vi "Coincidence vs trigger level.vi"(7 "Reset latch":refnum<vi>, 8 "error in (no error)":errorcluster, 10 "Set VTrig":refnum<vi>, 11 "VTrig mV":refnum<vi>) -> (0 "Error out":errorcluster)   [LabVIEW 2016]
uses:
  <vilib>/Platform/TimedLoop/XDataNode/timing_clust.ctl
  <vilib>/Platform/TimedLoop/XDataNode/nitl_modes.ctl
  <vilib>/Platform/TimedLoop/XDataNode/wakeup.ctl
  <vilib>/platform/TimedLoop/XDataNode/XDataNode.xnode
  <vilib>/Platform/TimedLoop/XDataNode/XDNodeRunTimeDep.lvlib
  <vilib>/Analysis/NI_AALBase.lvlib
panel:
  out "Previous trigger level":dbl
  out "Trigger level increment":dbl
  out "Datapoints":i32
  out "Level number":i32
  out "Current\n trigger level":dbl
  in  "Datapoints per level":i32
  in  "finish level":bool
  in  "Recommended at 25C":bool
  in  "MPPC Bias":dbl
  in  "ROB ID":i32
  in  "MPPC Serial number":i32
  in  "Scintillator ID":i32
  in  "Data":i32[](array[numeric])
  out "Command Queue":string[](array[string])
  in  "stop":bool
  out "Histogram Graph":T1(graph)
  out "Waveform Chart":dbl(graph)
  in  "base path":path=path "C:/Users/install/Google Drive/CRT/Labview/CRT Controller Folder/VIs/Data taking/test2"
  in  "Levels":i32
  in  "Range min":i32 format="%.0f  mV"
  in  "Range max":i32 format="%.0f mV"
  in  "Begin characterization":bool
  in  "Period":i32=1000 format="%.0f ms"
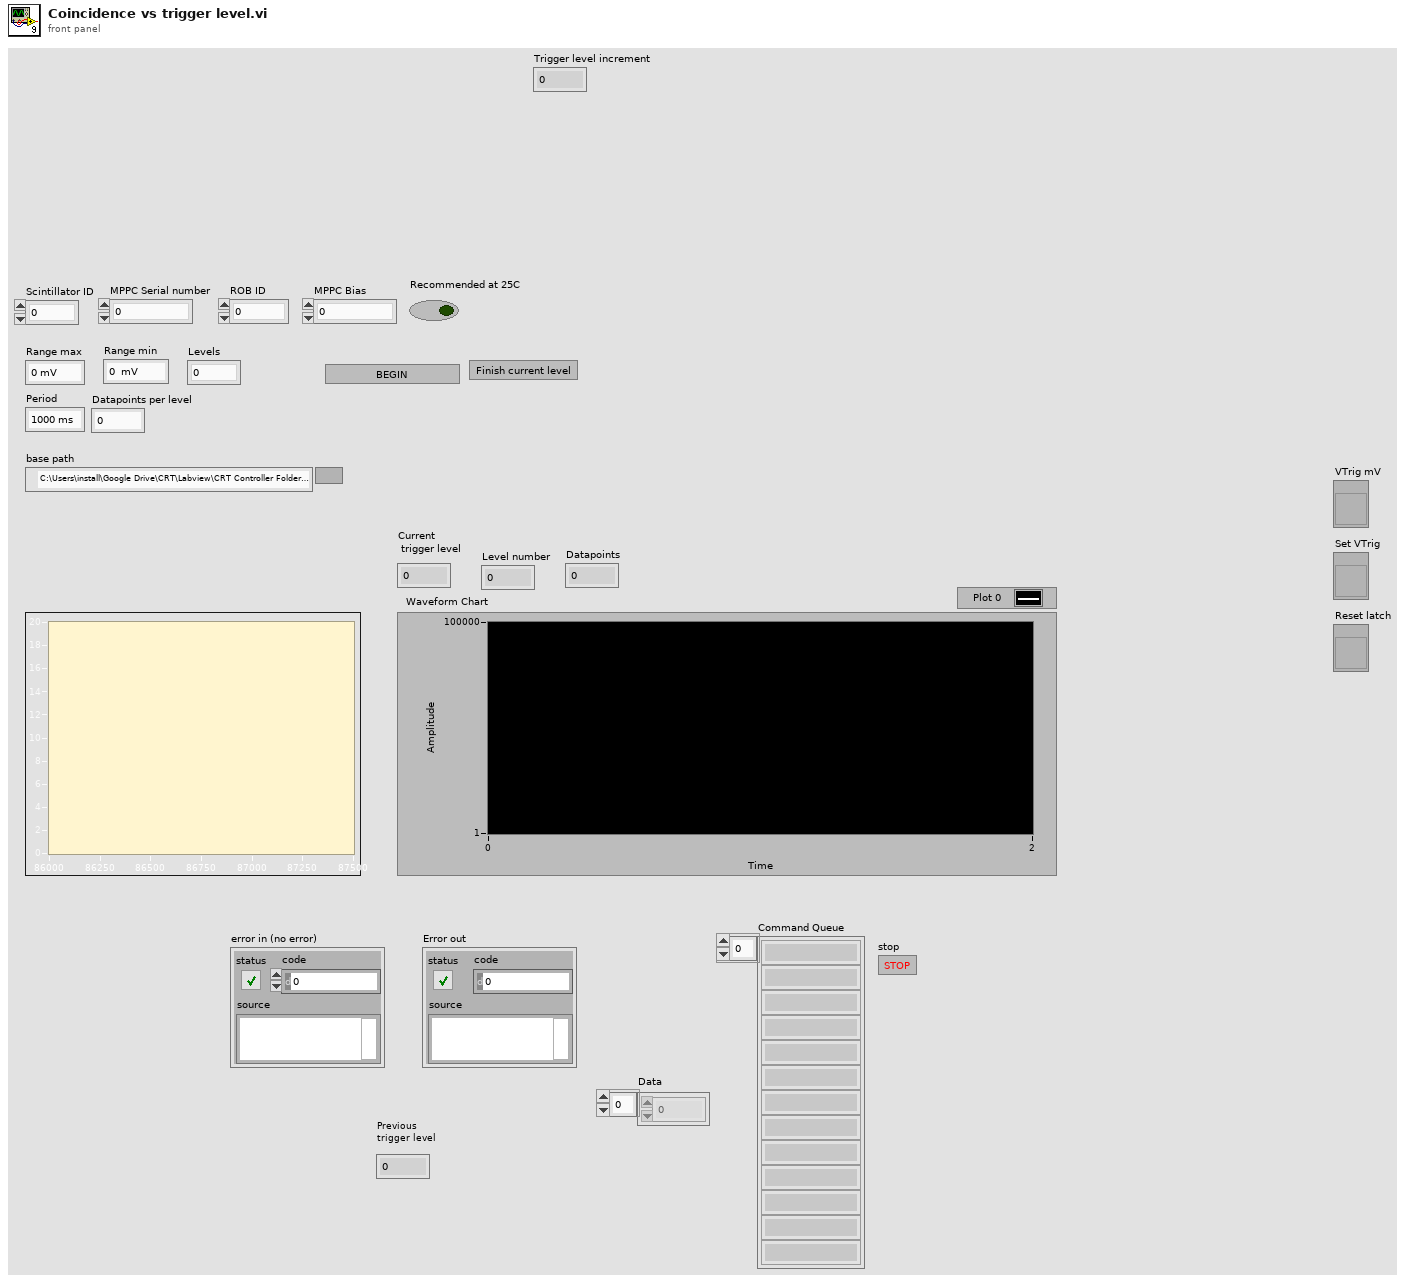
[diagram p1: front panel]
types:
  T1 = cluster{"X Values":dbl[], "Histogram: h(x)":i32[]}
  T2 = enum16{"open", "replace", "create", "open or create", "replace or create", "replace or create with confirmation"}
  T3 = enum16{"Reset", "ReadAndReset", "Read", "Add", "Init"}
  T4 = typedef "XDNodeRunTimeDep.lvlib/timing_clust.ctl" = cluster{"Expected End [f-1]":u64, "Actual End [f-1]":u64, "Finished Late? [f-1]":bool, "Expected End [i-1]":u64, "Actual End [i-1]":u64, "Finished Late? [i-1]":bool, "Expected Start [i]":u64, "Actual Start [i]":u64, "Expected Start [f]":u64, "Actual Start [f]":u64, "Source Name":string, "Structure Name":string, "Period":i64, "Deadline":i64, "Offset":i64, "Start":i64, "Priority":i32, "Timeout":i32, "Mode":T5, "Wakeup Reason":T6, "Error":errorcluster, "Source Type":string, "Secondary Source Type":string, "Global End Time":u64, "Global Start Time":u64, "Frame Duration":u64, "Iteration Duration":u64, "Assigned CPU":i32, "I/O Scan Engine Mode":u32}
  T5 = typedef "XDNodeRunTimeDep.lvlib/nitl_modes.ctl" = enum32{"No Change", "Process missed periods, maintain original phase", "Discard missed periods, maintain original phase", "Process missed periods, ignore original phase", "Discard missed periods, ignore original phase"}
  T6 = typedef "XDNodeRunTimeDep.lvlib/wakeup.ctl" = enum32{"Normal", "Aborted", "Asynchronous wakeup", "Timing source error", "Timed loop error", "Timeout"}
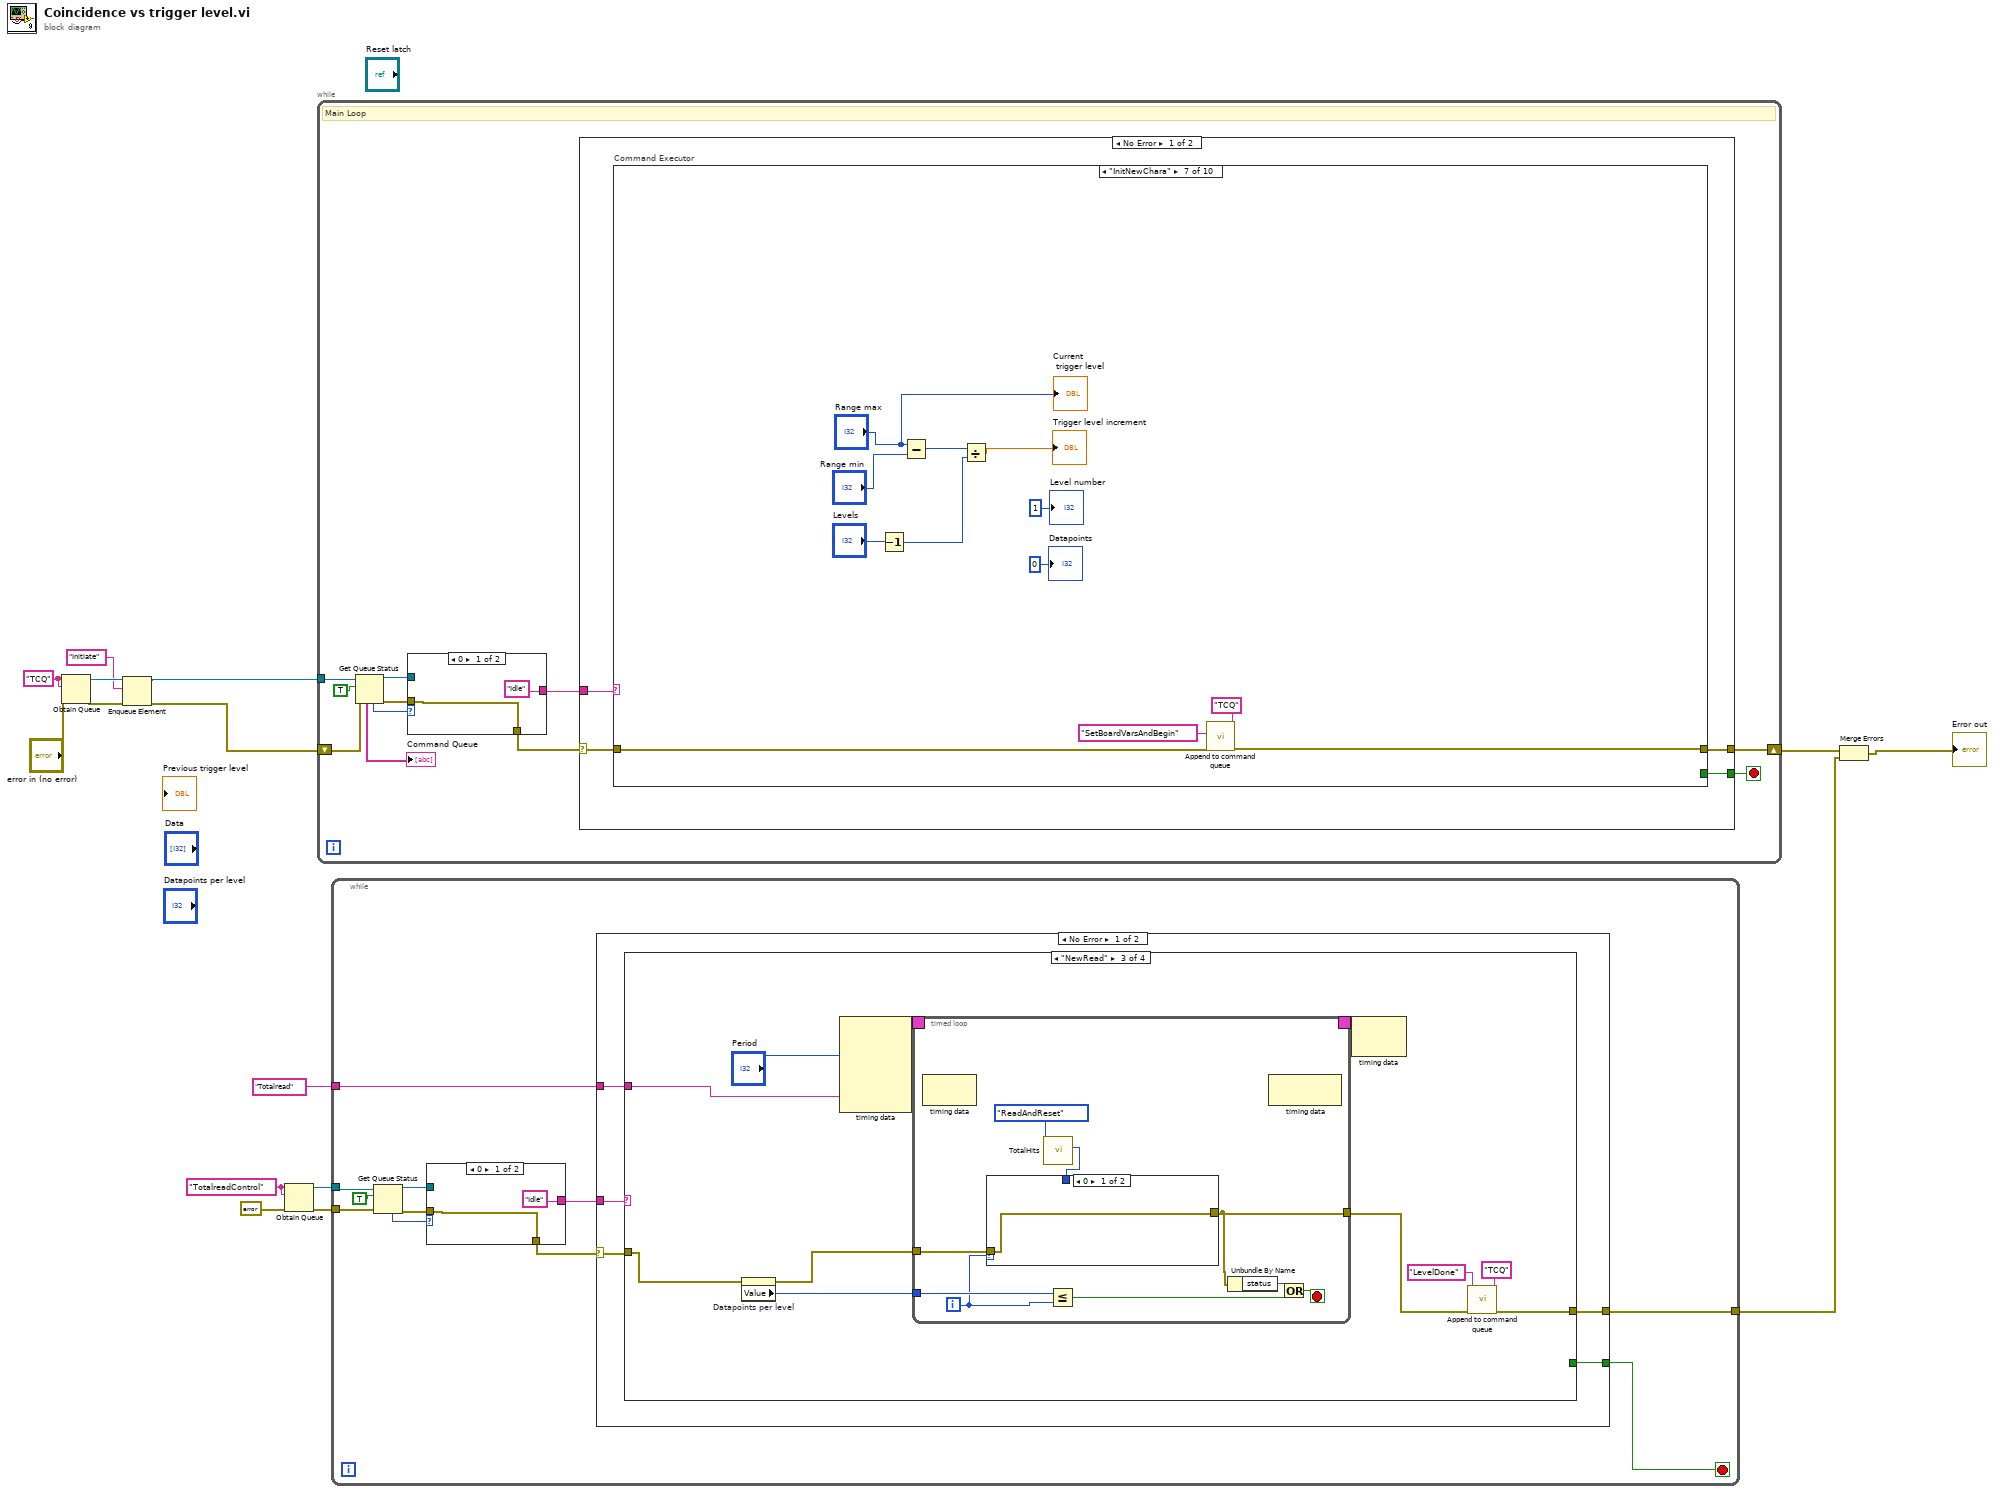
[diagram p0: block diagram]
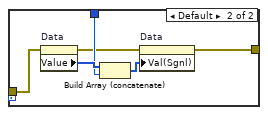
[diagram p4: hidden frame]
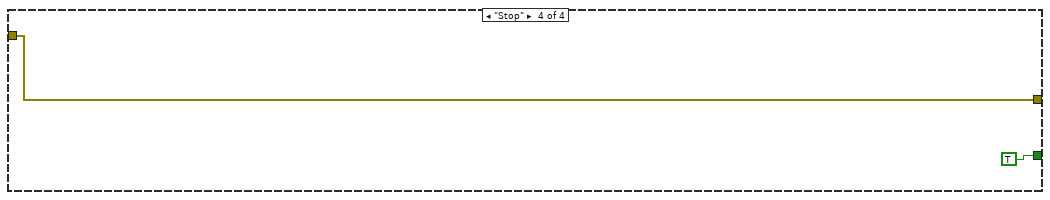
[diagram p5: hidden frame]
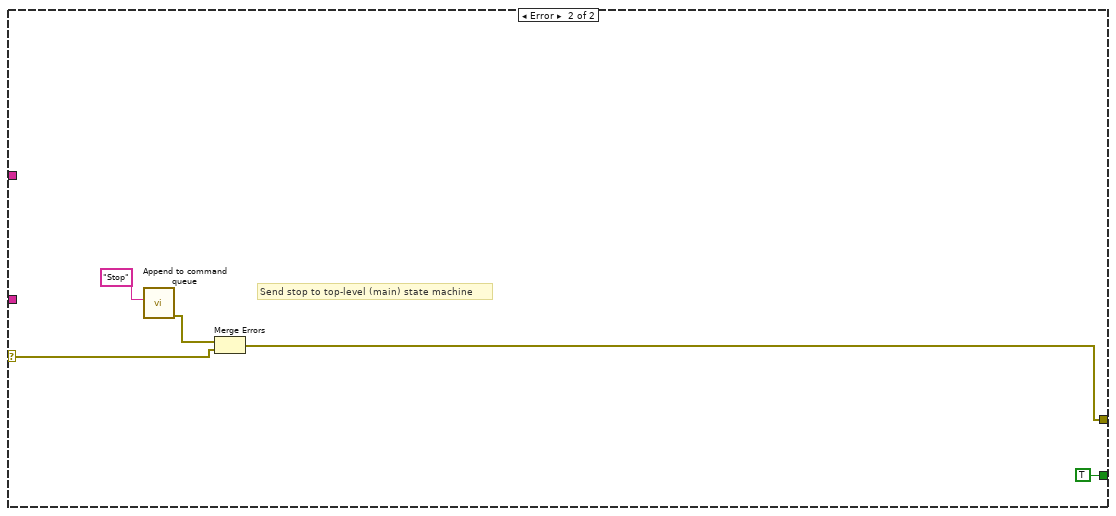
[diagram p6: hidden frame]
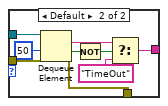
[diagram p7: hidden frame]
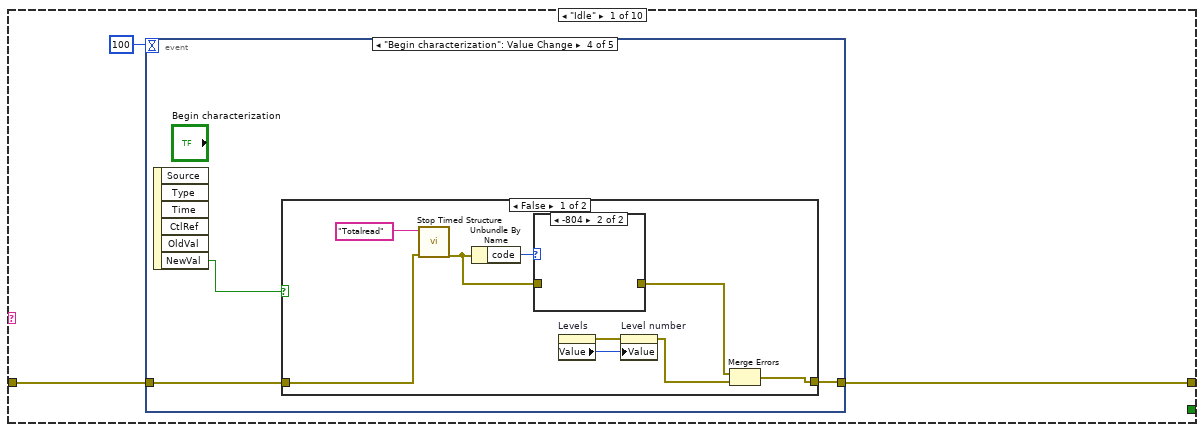
[diagram p8: hidden frame]
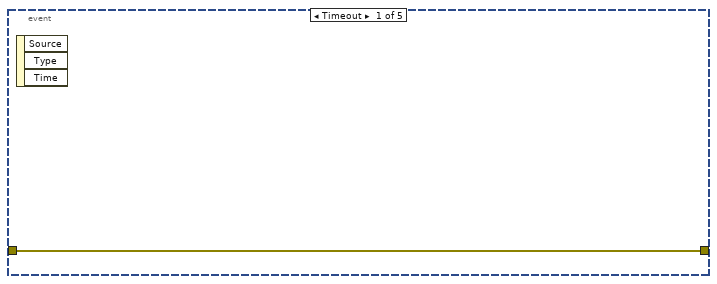
[diagram p9: hidden frame]
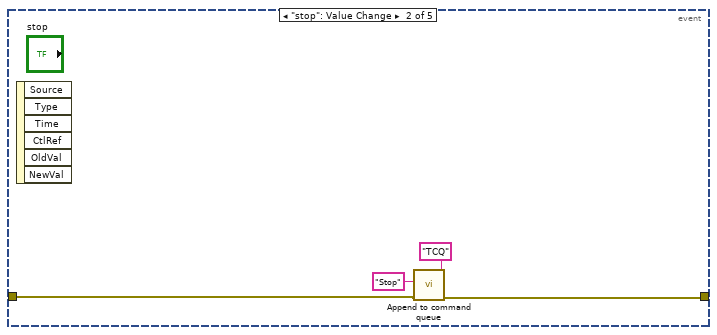
[diagram p10: hidden frame]
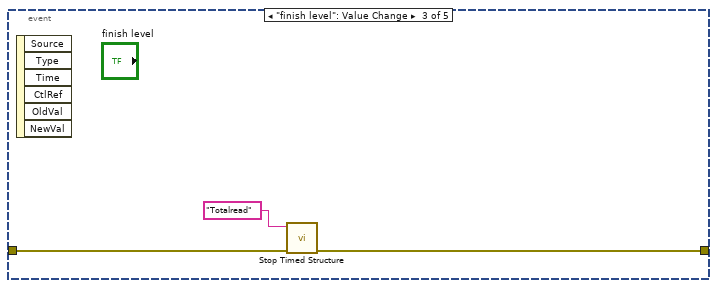
[diagram p11: hidden frame]
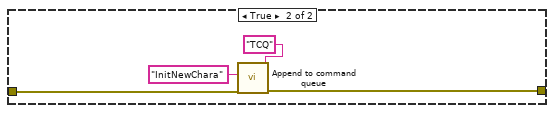
[diagram p13: hidden frame]
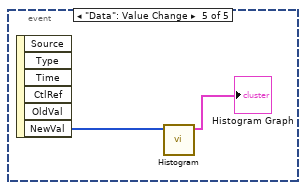
[diagram p14: hidden frame]
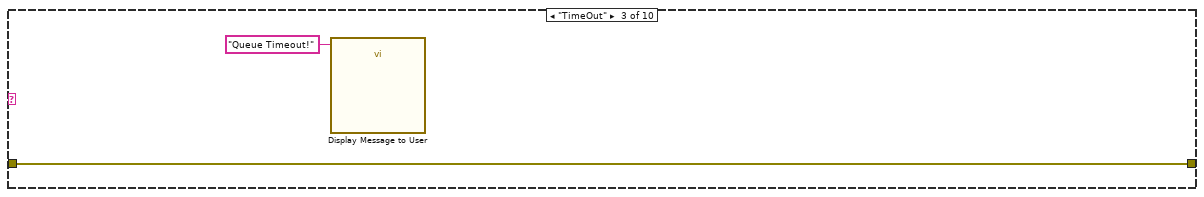
[diagram p16: hidden frame]
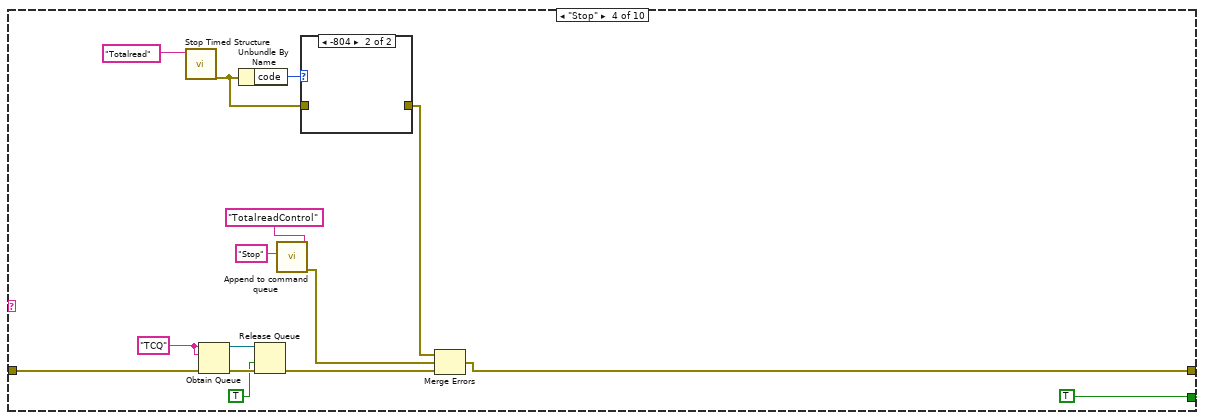
[diagram p17: hidden frame]
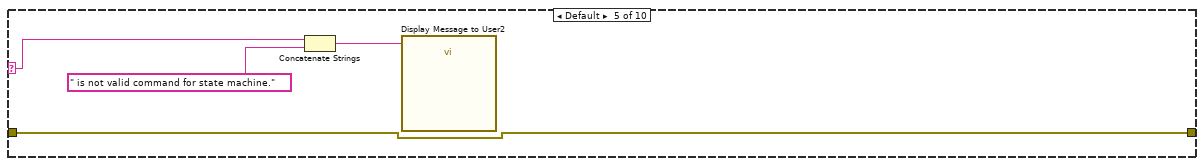
[diagram p19: hidden frame]
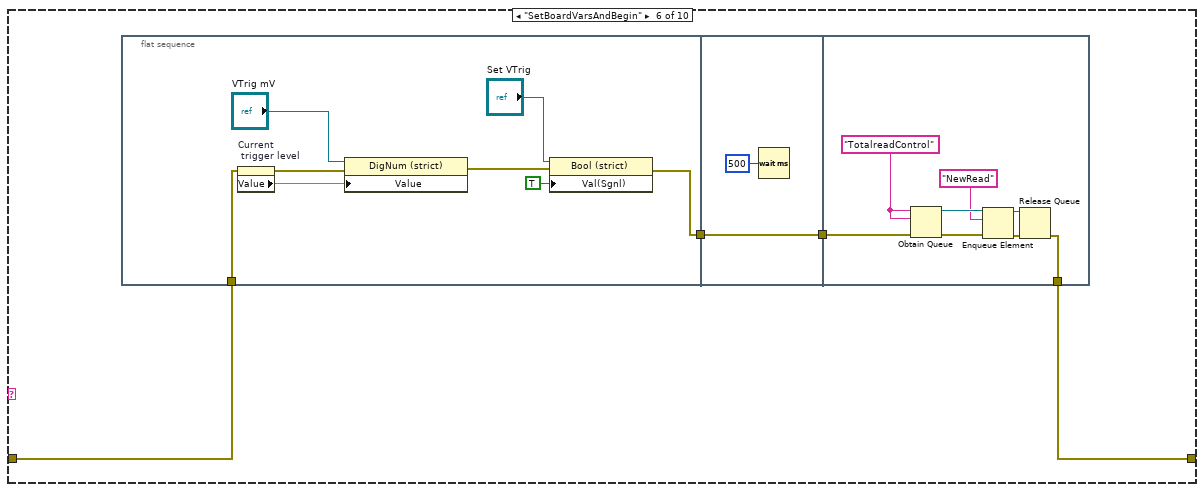
[diagram p20: hidden frame]
diagram:
  w7 = "TotalreadControl" ("name (unnamed)")
  w15 = "TCQ" ("name (unnamed)")
  n1 = Obtain Queue(name (unnamed)=w15, element data type=w15, error in (no error)="error in (no error)") -> (queue out=w13:refnum<queue>, error out=w11:errorcluster)  [unwired: 2 in, 1 out]
  n2 = Enqueue Element(queue=w13, element="Initiate", error in (no error)=w11) -> (queue out=w4:refnum<queue>, error out=w10:errorcluster)  [unwired: 1 in, 1 out]
  n3 = Obtain Queue(name (unnamed)=w7, element data type=w7, error in (no error)=errorcluster {"status"=FALSE, "code"=0, "source"=""}) -> (queue out=w6:refnum<queue>, error out=w5:errorcluster)  [unwired: 2 in, 1 out]
  n4 = while {
    tunnel: w4 -> [w22]
    shift-right: [w18] -> w3
    shift-left: w10 -> [w19]
    stop <- w17 stop-if-true
    # "Main Loop"
    n5 = Get Queue Status(queue=w22, return elements? (F)=TRUE, error in (no error)=w19) -> (queue out=w25:refnum<queue>, error out=w24:errorcluster, # elements in queue=w26:i32, elements=→"Command Queue":string[])  [unwired: 4 out]
    n6 = case shown="0" w26 {
      tunnel: ["Idle" ("element") w254] -> w20
      tunnel: w25 -> [_ w260]
      tunnel: w24 -> [w250 w259]
      tunnel: [w250 w253] -> w16
      frame 0 {
      }
      frame Default {
        n7 = Dequeue Element(queue=w260, timeout in ms (-1)=50, error in (no error)=w259) -> (element=w258:string, timed out?=w257:bool, error out=w253:errorcluster)  [unwired: 1 out]
        n8 = Not(x=w257) -> (.not. x?=w256:bool)
        n9 = Select(t=w258, s=w256, f="TimeOut") -> (s? t:f=w254:string)
      }
    }
    n10 = case shown="No Error" w16 {
      selector: w16 -> [w27 w242]
      tunnel: w20 -> [w30 _]
      tunnel: [w29 w241] -> w18
      tunnel: [w28 TRUE] -> w17
      frame No Error {
        n11 = case "Command Executor" shown="\"InitNewChara\"" w30 {
          selector: w30 -> [_ _ _ _ w81 _ _ _ _ _]
          tunnel: [w31 w61 w62 w64 w80 w84 w109 w125 w162 w227] -> w29
          tunnel: w27 -> [w32 w61 w62 w73 w80 w87 w110 w127 w164 w229]
          tunnel: [_ _ _ TRUE _ _ _ _ _ _] -> w28
          frame "Idle" {
            n12 = event shown="[3] \"Begin characterization\": Value Change" {
              selector: _ -> [_ _ _ _ _]
              dyn-events: _ -> [_ _ _ _ _]
              timeout: 100 -> [_ _ _ _ _]
              tunnel: w32 -> [w34 w38 w41 w44 _]
              tunnel: [w34 w37 w40 w43 _] -> w31
              event Timeout {
                n13 = event-data() -> ()  [unwired: 1 in, 3 out]
              }
              event "stop": Value Change {
                n14 = event-data() -> ()  [unwired: 1 in, 6 out]
                n15 = call "Append to command queue.vi"("Name (CommandQueue)"="TCQ", "error in (no error)"=w38, "Single command"="Stop") -> ("error out"=w37:errorcluster)  [unwired: 8 in]
              }
              event "finish level": Value Change {
                n16 = event-data() -> ()  [unwired: 1 in, 6 out]
                n17 = call <vilib>:"Stop Timed Structure.vi"("error in (no error)"=w41, "name"="Totalread" ("Structure Name")) -> ("error out"=w40:errorcluster)  [unwired: 9 in]
              }
              event "Begin characterization": Value Change {
                n18 = event-data() -> ("NewVal"=w42:bool)  [unwired: 1 in, 5 out]
                n19 = case shown="False" w42 {
                  tunnel: w44 -> [w48 w57]
                  tunnel: [w46 w56] -> w43
                  frame False {
                    n20 = call <vilib>:"Stop Timed Structure.vi"("error in (no error)"=w48, "name"="Totalread" ("Structure Name")) -> ("error out"=w49:errorcluster)  [unwired: 9 in]
                    n21 = Unbundle By Name(w49) -> ("code"=w50:i32)
                    n22 = case shown="-804" w50 {
                      tunnel: w49 -> [w54 _]
                      tunnel: [w54 _] -> w45
                      frame Default {
                      }
                      frame -804 {
                      }
                    }
                    n23 = property on="Levels" class="DigNum (strict)"() -> (error out=w52:errorcluster, "Value"=w53:i32)  [unwired: 2 in, 1 out]
                    n24 = property on="Level number" class="DigNum (strict)"(error in=w52, "Value"=w53) -> (error out=w47:errorcluster)  [unwired: 1 in, 1 out]
                    n25 = Merge Errors(w45, w47) -> (w46:errorcluster)
                  }
                  frame True {
                    n26 = call "Append to command queue.vi"("Name (CommandQueue)"="TCQ", "error in (no error)"=w57, "Single command"="InitNewChara") -> ("error out"=w56:errorcluster)  [unwired: 8 in]
                  }
                }
              }
              event "Data": Value Change {
                n27 = event-data() -> ("NewVal"=w59:i32[])  [unwired: 1 in, 5 out]
                n28 = call <vilib>:"Histogram.vi"("X"=w59) -> ("Histogram Graph"=→"Histogram Graph":T1)  [unwired: 7 in, 3 out]
              }
            }
          }
          frame "Initiate" {
          }
          frame "TimeOut" {
            n29 = call "Display Message to User"("Message"="Queue Timeout!" ("string")) -> ()  [unwired: 9 in, 2 out]
          }
          frame "Stop" {
            w74 = "TCQ" ("name (unnamed)")
            n30 = call <vilib>:"Stop Timed Structure.vi"("name"="Totalread" ("Structure Name")) -> ("error out"=w66:errorcluster)  [unwired: 10 in]
            n31 = Obtain Queue(name (unnamed)=w74, element data type=w74, error in (no error)=w73) -> (queue out=w77:refnum<queue>, error out=w76:errorcluster)  [unwired: 2 in, 1 out]
            n32 = Unbundle By Name(w66) -> ("code"=w69:i32)
            n33 = Release Queue(queue=w77, force destroy? (F)=TRUE, error in (no error)=w76) -> (error out=w67:errorcluster)  [unwired: 2 out]
            n34 = call "Append to command queue.vi"("Name (CommandQueue)"="TotalreadControl", "Single command"="Stop") -> ("error out"=w68:errorcluster)  [unwired: 9 in]
            n35 = case shown="-804" w69 {
              tunnel: w66 -> [w79 _]
              tunnel: [w79 _] -> w65
              frame Default {
              }
              frame -804 {
              }
            }
            n36 = Merge Errors(w65, w68, w67) -> (w64:errorcluster)
          }
          frame Default {
            n37 = Concatenate Strings(w81, " is not valid command for state machine." ("string")) -> (w82:string)
            n38 = call "Display Message to User2"("Message"=w82) -> ()  [unwired: 9 in, 2 out]
          }
          frame "SetBoardVarsAndBegin" {
            n39 = flat-sequence {
              tunnel: w87 -> [w89]
              tunnel: [w88] -> w86
              tunnel: w86 -> [w96]
              tunnel: [w96] -> w85
              tunnel: w85 -> [w100]
              tunnel: [w99] -> w84
              frame #0 {
                n40 = property on="Current\n trigger level" class="DigNum (strict)"(error in=w89) -> (error out=w91:errorcluster, "Value"=w92:dbl)  [unwired: 1 in, 1 out]
                n41 = property class="DigNum (strict)"(reference="VTrig mV", error in=w91, "Value"=w92) -> (error out=w90:errorcluster)  [unwired: 1 out]
                n42 = property class="Bool (strict)"(reference="Set VTrig", error in=w90, "Val(Sgnl)"=TRUE ("Value (Signaling)")) -> (error out=w88:errorcluster)  [unwired: 1 out]
              }
              frame #1 {
                n43 = Wait (ms)(milliseconds to wait=u32 500) -> ()  [unwired: 1 out]
              }
              frame #2 {
                w101 = "TotalreadControl" ("name (unnamed)")
                n44 = Obtain Queue(name (unnamed)=w101, element data type=w101, error in (no error)=w100) -> (queue out=w105:refnum<queue>, error out=w104:errorcluster)  [unwired: 2 in, 1 out]
                n45 = Enqueue Element(queue=w105, element="NewRead", error in (no error)=w104) -> (queue out=w102:refnum<queue>, error out=w103:errorcluster)  [unwired: 1 in, 1 out]
                n46 = Release Queue(queue=w102, error in (no error)=w103) -> (error out=w99:errorcluster)  [unwired: 1 in, 2 out]
              }
            }
          }
          frame "InitNewChara" {
            n47 = Decrement(x="Levels") -> (x-1=w106:i32)
            n48 = Subtract(x="Range max", y="Range min") -> (x-y=w115:i32)
            n49 = Divide(x=w115, y=w106) -> (x/y=→"Trigger level increment":dbl)
            n50 = call "Append to command queue.vi"("Name (CommandQueue)"="TCQ", "error in (no error)"=w110, "Single command"="SetBoardVarsAndBegin") -> ("error out"=w109:errorcluster)  [unwired: 8 in]
            "Current\n trigger level" <- "Range max"
            "Level number" <- 1 ("Level number")
            "Datapoints" <- 0 ("Datapoints")
          }
          frame "LevelDone" {
            n51 = property on="Levels" class="DigNum (strict)"(error in=w127) -> (error out=w128:errorcluster, "Value"=w129:i32)  [unwired: 1 in, 1 out]
            n52 = property on="Level number" class="DigNum (strict)"(error in=w128) -> (error out=w122:errorcluster, "Value"=w130:i32)  [unwired: 1 in, 1 out]
            n53 = Equal?(x=w130, y=w129) -> (x = y?=w126:bool)
            n54 = call "Append to command queue.vi"("Name (CommandQueue)"="TCQ", "error in (no error)"=w122, "Single command"="SaveData") -> ("error out"=w119:errorcluster)  [unwired: 8 in]
            n55 = property on="Current\n trigger level" class="DigNum (strict)"(error in=w119) -> (error out=w120:errorcluster, "Value"=w121:dbl)  [unwired: 1 in, 1 out]
            n56 = property on="Previous trigger level" class="DigNum (strict)"(error in=w120, "Value"=w121) -> (error out=w118:errorcluster)  [unwired: 1 in, 1 out]
            n57 = case shown="False" w126 {
              tunnel: w118 -> [w136 w147]
              tunnel: [w133 w146] -> w125
              frame False {
                n58 = property on="Trigger level increment" class="DigNum (strict)"(error in=w136) -> (error out=w141:errorcluster, "Value"=w140:dbl)  [unwired: 1 in, 1 out]
                n59 = property on="Current\n trigger level" class="DigNum (strict)"(error in=w141) -> (error out=w138:errorcluster, "Value"=w131:dbl)  [unwired: 1 in, 1 out]
                n60 = Subtract(x=w131, y=w140) -> (x-y=w139:dbl)
                n61 = property on="Current\n trigger level" class="DigNum (strict)"(error in=w138, "Value"=w139) -> (error out=w137:errorcluster)  [unwired: 1 in, 1 out]
                n62 = property on="Level number" class="DigNum (strict)"(error in=w137) -> (error out=w142:errorcluster, "Value"=w144:i32)  [unwired: 1 in, 1 out]
                n63 = Increment(x=w144) -> (x+1=w143:i32)
                n64 = property on="Level number" class="DigNum (strict)"(error in=w142, "Value"=w143) -> (error out=w132:errorcluster)  [unwired: 1 in, 1 out]
                n65 = call "Append to command queue.vi"("Name (CommandQueue)"="TCQ", "error in (no error)"=w132, "Single command"="SetBoardVarsAndBegin") -> ("error out"=w133:errorcluster)  [unwired: 8 in]
              }
              frame True {
                n66 = call "Append to command queue.vi"("Name (CommandQueue)"="TCQ", "error in (no error)"=w147, "Single command"="Reset") -> ("error out"=w146:errorcluster)  [unwired: 8 in]
              }
            }
          }
          frame "SaveData" {
            w153 = "\t"
            n67 = control-ref of="Period"() -> (w203:refnum<vi>)
            n68 = control-ref of="Previous trigger level"() -> (w156:refnum<vi>)
            n69 = property class="DigNum (strict)"(reference=w203, error in=w164) -> (error out=w189:errorcluster, "Value"=w172:i32)  [unwired: 1 out]
            n70 = property class="DigNum (strict)"(reference=w156, error in=w189) -> (error out=w188:errorcluster, "Value"=w204:dbl)  [unwired: 1 out]
            n71 = property on="Data" class="Arr (strict)"(error in=w188) -> (error out=w187:errorcluster, "Value"=w171:i32[])  [unwired: 1 in, 1 out]
            n72 = property on="base path" class="Path"(error in=w164) -> (error out=w163:errorcluster, "Value"=w185:path)  [unwired: 1 in, 1 out]
            n73 = Build Path(base path=w185, name or relative path="Summary.csv") -> (appended path=w180:path)
            n74 = Number To Decimal String(number=w204) -> (decimal integer string=w168:string)  [unwired: 1 in]
            n75 = Number To Decimal String(number=w172) -> (decimal integer string=w155:string)  [unwired: 1 in]
            n76 = Open/Create/Replace File(file path (use dialog)=w180, error in=w163, operation (0:open)=T2."open") -> (refnum out=w183:refnum<file>, error out=w182:errorcluster)  [unwired: 3 in, 1 out]
            n77 = Unbundle By Name(w182) -> ("code"=w181:i32)
            n78 = Concatenate Strings(w168, "mV " ("string"), w155, "s.csv " ("string")) -> (w202:string)
            n79 = Array To Spreadsheet String(delimiter (Tab)="\r\n", array=w171, 3:"%d" ("format string")) -> (spreadsheet string=w195:string)
            n80 = Build Path(base path="base path", name or relative path=w202) -> (appended path=w207:path)
            n81 = call "Build header single level.vi"("Overvoltage"="MPPC Bias", "Recommended at 25C"="Recommended at 25C", "MPPC Serial number"="MPPC Serial number", "ROB ID"="ROB ID", "Scintillator ID"="Scintillator ID") -> ("Header"=w179:string)  [unwired: 6 in]
            n82 = case shown="7" w181 {
              tunnel: w183 -> [_ w226]
              tunnel: w182 -> [_ w225]
              tunnel: w180 -> [w218 _]
              tunnel: w179 -> [w213 _]
              tunnel: [w215 w221] -> w173
              tunnel: [w214 w220] -> w174
              frame 7 {
                n83 = Open/Create/Replace File(file path (use dialog)=w218, operation (0:open)=T2."create") -> (refnum out=w216:refnum<file>, error out=w217:errorcluster)  [unwired: 4 in, 1 out]
                n84 = Concatenate Strings(w213, "Trigger\tmean\tstandard deviation\tvariance\tpool size\tperiod" ("delimiter (Tab)"), "\r\n") -> (w211:string)
                n85 = Write to Text File(file (use dialog)=w216, text=w211, error in=w217) -> (refnum out=w215:refnum<file>, error out=w214:errorcluster)  [unwired: 1 in, 1 out]
              }
              frame Default {
                n86 = Get File Size(file=w226, error in=w225) -> (refnum out=w224:refnum<file>, size (in bytes)=w223:i64, 0:w222:errorcluster)
                n87 = Set File Position(offset (in bytes) (0)=w223, refnum=w224, error in=w222) -> (refnum out=w221:refnum<file>, error out=w220:errorcluster)  [unwired: 1 in]
              }
            }
            n88 = Concatenate Strings(w179, w195) -> (w192:string)
            n89 = Open/Create/Replace File(file path (use dialog)=w207, error in=w187, operation (0:open)=T2."open or create") -> (refnum out=w194:refnum<file>, error out=w193:errorcluster)  [unwired: 3 in, 1 out]
            n90 = call <vilib>:"Std Deviation and Variance.vi"("X"=w171) -> ("mean"=w157:dbl, "standard deviation"=w178:dbl, "variance"=w177:dbl)  [unwired: 1 in]
            "Waveform Chart" <- w157
            n91 = Array Size(array=w171) -> (size(s)=w170:i32)
            n92 = Build Array(w157, w178, w177) -> (w175:dbl[])
            n93 = Number To Decimal String(number=w170) -> (decimal integer string=w167:string)  [unwired: 1 in]
            n94 = Write to Text File(file (use dialog)=w194, text=w192, error in=w193) -> (refnum out=w191:refnum<file>, error out=w190:errorcluster)  [unwired: 1 in, 1 out]
            n95 = Array To Spreadsheet String(array=w175, 3:"%5.3f" ("format string")) -> (spreadsheet string=w152:string)  [unwired: 1 in]
            n96 = Close File(refnum=w191, error in=w190) -> (error out=w160:errorcluster)  [unwired: 1 out]
            n97 = Search/Split String(string=w152, search string/char (-)="\r\n") -> (substring before match=w150:string)  [unwired: 1 in, 2 out]
            n98 = Concatenate Strings(w168, w153, w150, w153, w167, w153, w155, "\r\n") -> (w169:string)
            n99 = Write to Text File(file (use dialog)=w173, text=w169, error in=w174) -> (refnum out=w165:refnum<file>, error out=w166:errorcluster)  [unwired: 1 in, 1 out]
            n100 = property on="Data" class="Arr (strict)"(error in=w160, "Value"=i32[] [] ("Data")) -> (error out=w159:errorcluster)  [unwired: 1 in, 1 out]
            n101 = Close File(refnum=w165, error in=w166) -> (error out=w161:errorcluster)  [unwired: 1 out]
            n102 = Merge Errors(w161, w159) -> (w162:errorcluster)
          }
          frame "Reset" {
            n103 = property on="Level number" class="DigNum (strict)"(error in=w229, "Value"=1 ("Level number")) -> (error out=w228:errorcluster)  [unwired: 1 in, 1 out]
            n104 = property on="Datapoints" class="DigNum (strict)"(error in=w228, "Value"=0 ("Datapoints")) -> (error out=w227:errorcluster)  [unwired: 1 in, 1 out]
          }
        }
      }
      frame Error {
        w244 = "TCQ" ("name (unnamed)")
        n105 = call <vilib>:"Stop Timed Structure.vi"("name"="Totalread" ("Structure Name")) -> ("error out"=w233:errorcluster)  [unwired: 10 in]
        n106 = Obtain Queue(name (unnamed)=w244, element data type=w244) -> (queue out=w247:refnum<queue>, error out=w246:errorcluster)  [unwired: 3 in, 1 out]
        n107 = Unbundle By Name(w233) -> ("code"=w234:i32)
        n108 = call "Append to command queue.vi"("Single command"="Stop") -> ("error out"=w239:errorcluster)  [unwired: 10 in]
        n109 = Release Queue(queue=w247, force destroy? (F)=TRUE, error in (no error)=w246) -> (error out=w243:errorcluster)  [unwired: 2 out]
        n110 = case shown="-804" w234 {
          tunnel: w233 -> [w249 _]
          tunnel: [w249 _] -> w232
          frame Default {
          }
          frame -804 {
          }
        }
        n111 = call "Append to command queue.vi"("Name (CommandQueue)"="TotalreadControl", "Single command"="Stop") -> ("error out"=w236:errorcluster)  [unwired: 9 in]
        n112 = Merge Errors(w232, w236, w239, w243, w242) -> (w241:errorcluster)
      }
    }
  }
  n113 = while {
    tunnel: "Totalread" ("Structure Name") -> [w271]
    tunnel: w6 -> [w266]
    tunnel: w5 -> [w265]
    tunnel: [w262] -> w2
    stop <- w261 stop-if-true
    n114 = Get Queue Status(queue=w266, return elements? (F)=TRUE, error in (no error)=w265) -> (queue out=w269:refnum<queue>, error out=w268:errorcluster, # elements in queue=w270:i32)  [unwired: 5 out]
    n115 = case shown="0" w270 {
      tunnel: ["Idle" ("element") w324] -> w264
      tunnel: w269 -> [_ w330]
      tunnel: w268 -> [w320 w329]
      tunnel: [w320 w323] -> w263
      frame 0 {
      }
      frame Default {
        n116 = Dequeue Element(queue=w330, timeout in ms (-1)=50, error in (no error)=w329) -> (element=w328:string, timed out?=w327:bool, error out=w323:errorcluster)  [unwired: 1 out]
        n117 = Not(x=w327) -> (.not. x?=w326:bool)
        n118 = Select(t=w328, s=w326, f="TimeOut") -> (s? t:f=w324:string)
      }
    }
    n119 = case shown="No Error" w263 {
      selector: w263 -> [w274 w317]
      tunnel: w271 -> [w276 _]
      tunnel: w264 -> [w275 _]
      tunnel: [w273 w316] -> w262
      tunnel: [w272 TRUE] -> w261
      frame No Error {
        n120 = case shown="\"NewRead\"" w275 {
          tunnel: w276 -> [_ _ w289 _]
          tunnel: [w277 w278 w288 w314] -> w273
          tunnel: w274 -> [w277 w278 w287 w314]
          tunnel: [_ _ _ TRUE] -> w272
          frame "TimeOut" {
          }
          frame Default {
          }
          frame "NewRead" {
            n121 = property on="Datapoints per level" class="DigNum (strict)"(error in=w287) -> (error out=w280:errorcluster, "Value"=w279:i32)  [unwired: 1 in, 1 out]
            n122 = node-c288("Period", w289) -> (w286:T4)  [unwired: 3 in]
            n123 = timed-loop {
              timing: w286 -> [_]
              timing-out: [_] -> w285
              tunnel: w280 -> [w296]
              tunnel: [w294] -> w281
              tunnel: w279 -> [w295]
              i -> [w290]
              stop <- w291 stop-if-true
              n124 = node-c288() -> ()  [unwired: 1 in, 1 out]
              n125 = call "TotalHits.vi"("Action"=T3."ReadAndReset") -> ("Result"=w297:u64)  [unwired: 10 in]
              n126 = case shown="0" w290 {
                tunnel: w297 -> [_ w304]
                tunnel: w296 -> [w299 w301]
                tunnel: [w299 w300] -> w294
                frame 0 {
                }
                frame Default {
                  n127 = property on="Data" class="Arr (strict)"(error in=w301) -> (error out=w302:errorcluster, "Value"=w305:i32[])  [unwired: 1 in, 1 out]
                  n128 = Build Array (concatenate)(w305, w304) -> (w303:u64[])
                  n129 = property on="Data" class="Arr (strict)"(error in=w302, "Val(Sgnl)"=w303) -> (error out=w300:errorcluster)  [unwired: 1 in, 1 out]
                }
              }
              n130 = Less Or Equal?(x=w295, y=w290) -> (x <= y?=w292:bool)
              n131 = Unbundle By Name(w294) -> ("status"=w293:bool)
              n132 = node-c288() -> ()  [unwired: 1 in, 1 out]
              n133 = Or(x=w293, y=w292) -> (x .or. y?=w291:bool)
            }
            n134 = node-c288(w285) -> ()  [unwired: 1 out]
            n135 = call "Append to command queue.vi"("Name (CommandQueue)"="TCQ" ("name (unnamed)"), "error in (no error)"=w281, "Single command"="LevelDone") -> ("error out"=w288:errorcluster)  [unwired: 8 in]
          }
          frame "Stop" {
          }
        }
      }
      frame Error {
        # "Send stop to top-level (main) state machine"
        n136 = call "Append to command queue.vi"("Single command"="Stop") -> ("error out"=w318:errorcluster)  [unwired: 10 in]
        n137 = Merge Errors(w318, w317) -> (w316:errorcluster)
      }
    }
  }
  n138 = Merge Errors(w3, w2) -> (→"Error out":errorcluster)
